vi "pageChefProjet.vi"(0 "role":string, 1 "Choix":i16(ring) items=["admin", "alexis", "julien", "florian", "saco", "aaaaa"], 2 "Projet":i16(ring) items=["Meuble"], 3 "id_personnel_connect":string, 4 "OK Button":bool, 5 "Action":i16(ring) items=["Supprimer un employé", "Ajouter un employé"]) -> (6 "Table Control":string[][](table), 7 "liste_projet":string[](array[string]), 8 "liste_personnel":string[](array[string]))   [LabVIEW 2024]
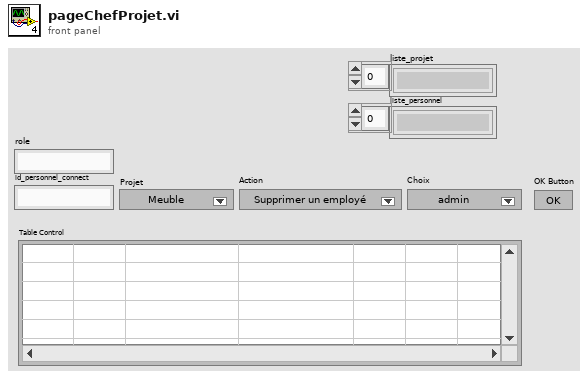
[diagram p1: front panel]
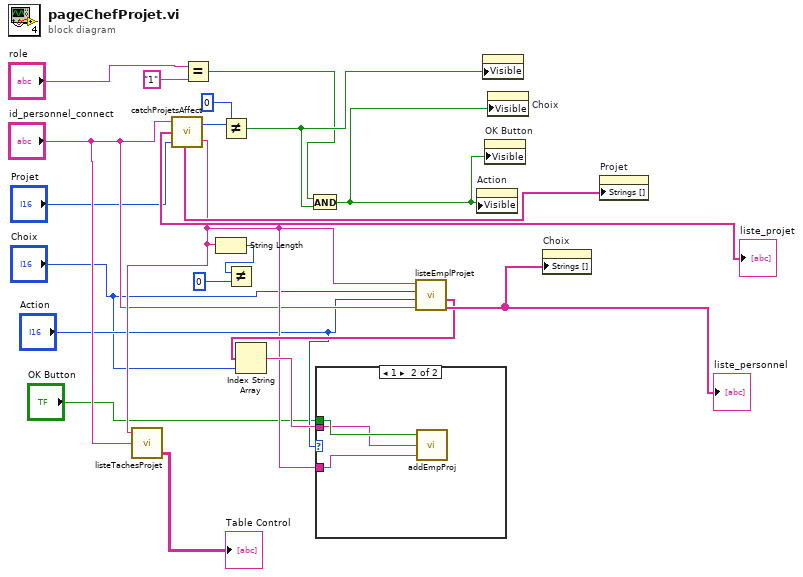
[diagram p0: block diagram]
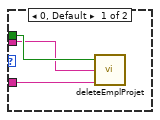
[diagram p2: hidden frame]
diagram:
  n1 = call "catchProjetsAffect.vi"("Choix"="Projet", "Id personnel"="id_personnel_connect") -> ("String"=w9:string, "size(s)"=w15:i32, "subarray"=w19:string[])
  "liste_projet" <- w19
  n2 = call "listeTachesProjet.vi"("Id Personnel"="id_personnel_connect", "Id Projet"=w9) -> ("Table Control"=→"Table Control":string[][])
  n3 = Equal?(x="role", y="1") -> (x = y?=w12:bool)
  n4 = String Length(string=w9) -> (length=w17:i32)
  n5 = Not Equal?(x=0, y=w15) -> (x != y?=w13:bool)
  n6 = Not Equal?(x=w17, y=0) -> ()  [unwired: 1 out]
  n7 = And(x=w12, y=w13) -> (x .and. y?=w3:bool)
  n8 = call "listeEmplProjet.vi"("id personnel courant"="id_personnel_connect", "Suppr/Delete"="Action", "Choix"="Choix", "Id projet"=w9) -> ("name"=w20:string[], "id"=w11:string[])  [unwired: 2 out]
  "liste_personnel" <- w20
  n9 = Index String Array(1:"Choix", 2:w11) -> (0:w10:string)  [unwired: 1 in]
  n10 = case shown="1" "Action" {
    tunnel: w10 -> [w22 w25]
    tunnel: "OK Button" -> [w23 w26]
    tunnel: w9 -> [w21 w24]
    frame 0, Default {
      n11 = call "deleteEmplProjet.vi"("id projet"=w21, "Id Personnel"=w22, "OK Button"=w23) -> ()
    }
    frame 1 {
      n12 = call "addEmpProj.vi"("Identifiant Projet"=w24, "Identifiant Emp"=w25, "OK Button"=w26) -> ()
    }
  }
  n13 = property on="Action" class="Ring (strict)"("Visible"=w3) -> ()  [unwired: 2 in, 2 out]
  n14 = property on="Projet" class="Ring (strict)"("Visible"=w13) -> ()  [unwired: 2 in, 2 out]
  n15 = property on="OK Button" class="Bool"("Visible"=w3) -> ()  [unwired: 2 in, 2 out]
  n16 = property on="Choix" class="Ring (strict)"("Visible"=w3) -> ()  [unwired: 2 in, 2 out]
  n17 = property on="Choix" class="Ring (strict)"("Strings []"=w20) -> ()  [unwired: 2 in, 2 out]
  n18 = property on="Projet" class="Ring (strict)"("Strings []"=w19) -> ()  [unwired: 2 in, 2 out]
